vi "find_read_width_2017.10.24.vi"(10 "timetags":u32[][](array[numeric]), 11 "T1_parameters":T2) -> (2 "hist_q1-read_width":T1, 3 "proposed_read_width_us":dbl)   [LabVIEW 2014]
uses:
  <vilib>/Analysis/1siggen.llb/Ramp Pattern by Delta.vi
  <vilib>/Analysis/NI_AALBase.lvlib
panel:
  in  "step_size_us":dbl=0.01
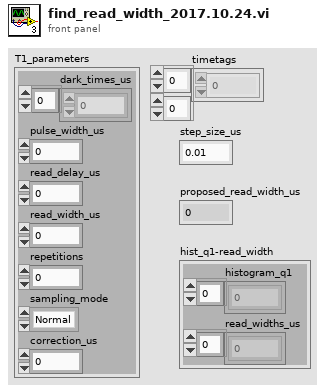
[diagram p1: front panel]
types:
  T1 = cluster{"read_widths_us":dbl[], "histogram_q1":i32[]}
  T2 = cluster{"dark_times_us":dbl[], "pulse_width_us":dbl, "read_delay_us":dbl, "read_width_us":dbl, "repetitions":i32, "sampling_mode":enum16{"Normal", "Sweep"}, "correction_us":dbl}
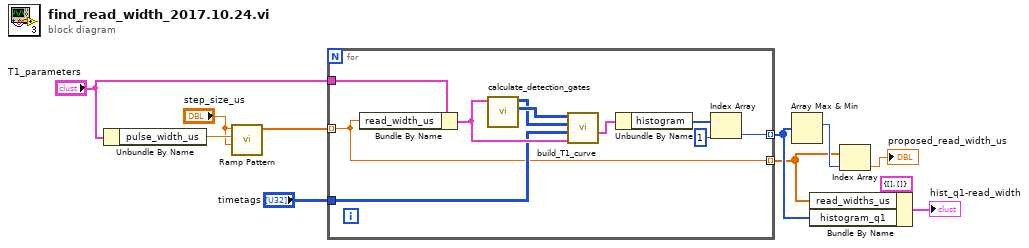
[diagram p0: block diagram]
diagram:
  n1 = Unbundle By Name("T1_parameters") -> ("pulse_width_us"=w11:dbl)
  n2 = call-poly <vilib>:"Ramp Pattern.vi"("start"="step_size_us", "end"=w11, "delta"="step_size_us") -> ("Ramp Pattern"=w9:dbl[])  [unwired: 6 in, 2 out]
  n3 = for {
    tunnel: w9 -> [w12] mode=indexing
    tunnel: "T1_parameters" -> [w15]
    tunnel: "timetags" -> [w14]
    tunnel: [w13] -> w3 mode=indexing
    tunnel: [w12] -> w2 mode=indexing
    n4 = Bundle By Name(cluster=w15, "read_width_us"=w12) -> (w21:T2)
    n5 = call "calculate_detection_gates.vi"("T1_parameters"=w21) -> ("start_read"=w17:u32[][], "stop_read"=w16:u32[][])  [unwired: 9 in]
    n6 = call "build_T1_curve.vi"("T1_parameters"=w21, "timetags"=w14, "stop_read"=w16, "start_read"=w17) -> ("histogram"=w20:cluster{"q_photons":i32[], "histogram":i32[]})  [unwired: 5 in, 2 out]
    n7 = Unbundle By Name(w20) -> ("histogram"=w18:i32[])
    n8 = Index Array(array=w18, index=1) -> (element=w13:i32)
  }
  n9 = Array Max & Min(array=w3) -> (max index (indices)=w6:i32)  [unwired: 3 out]
  n10 = Bundle By Name(cluster=T1 {"read_widths_us"=[], "histogram_q1"=[]} ("hist1-read_width"), "read_widths_us"=w2, "histogram_q1"=w3) -> (→"hist_q1-read_width":T1)
  n11 = Index Array(array=w2, index=w6) -> (element=→"proposed_read_width_us":dbl)
